vi "Shutdown Daemon.vi"(8 "error in (no error)":errorcluster, 11 "serial slave in":refnum<class "Serial Slave.lvclass">) -> (0 "error out":errorcluster)   [LabVIEW 2017, in "SubVIs.lvlib" / "Serial Slave.lvclass"]
doc: "This provides an interface for the slave to shut down its protocol daemon."
uses:
  <vilib>/Modbus/subvis/Protocol/Serial/Serial Slave/Serial Slave.lvclass
  <vilib>/Modbus/subvis/Protocol/Serial/Serial Slave/Serial Slave.lvclass/Serial Slave.ctl
  <vilib>/Modbus/subvis/Protocol/Interfaces/Network Slave/Network Slave.lvclass
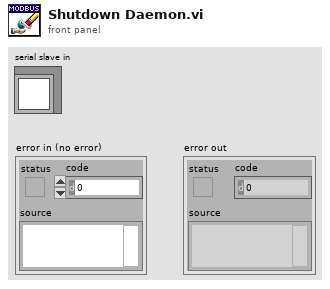
[diagram p1: front panel]
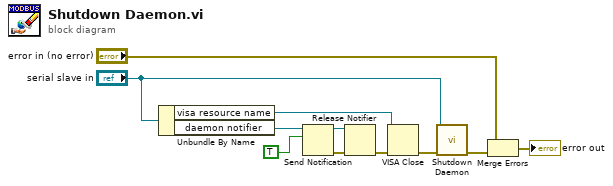
[diagram p0: block diagram]
diagram:
  n1 = Unbundle By Name("serial slave in") -> ("visa resource name"=w1:refnum<visa-resource-name>, "daemon notifier"=w8:refnum<notifier>)
  n2 = Send Notification(notification=TRUE, notifier=w8) -> (notifier out=w10:refnum<notifier>, error out=w9:errorcluster)  [unwired: 1 in]
  n3 = Release Notifier(notifier=w10, error in (no error)=w9) -> (error out=w6:errorcluster)  [unwired: 1 in, 2 out]
  n4 = VISA Close(VISA resource name=w1, error in (no error)=w6) -> (error out=w2:errorcluster)
  n5 = call-parent "Shutdown Daemon.vi"("error in (no error)"=w2, "network slave in"="serial slave in") -> ("error out"=w5:errorcluster)  [unwired: 9 in]
  n6 = Merge Errors("error in (no error)", w5) -> (→"error out":errorcluster)
